vi "Analyse.vi"(8 "error in (no error)":errorcluster, 10 "ImageData":T1, 11 "AbsorptionAnalyser in":refnum<class "AbsorptionAnalyserNTU.lvclass">) -> (0 "error out":errorcluster, 3 "AbsorptionAnalyser out":refnum<class "AbsorptionAnalyserNTU.lvclass">)   [LabVIEW 2011, in "AbsorptionAnalyserNTU.lvclass"]
uses:
  AbsorptionAnalyserNTU.lvclass
  AbsorptionAnalyserNTU.lvclass/AbsorptionAnalyserNTU.ctl
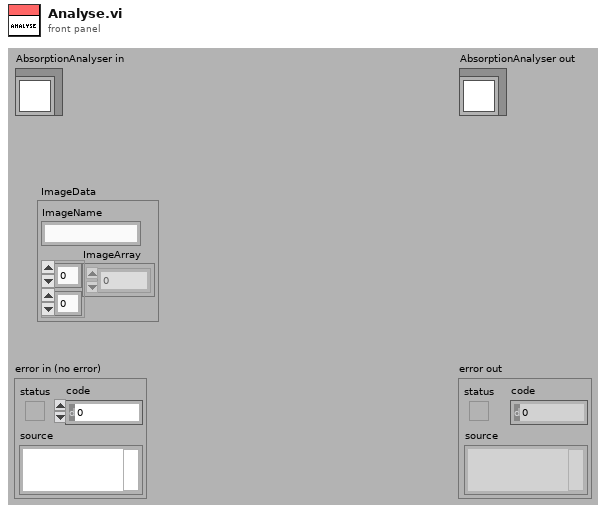
[diagram p1: front panel]
types:
  T1 = cluster{"ImageName":string, "ImageArray":sgl[][]}
  T2 = cluster{"ImageName":string, "ImageArray":sgl[][]}[]
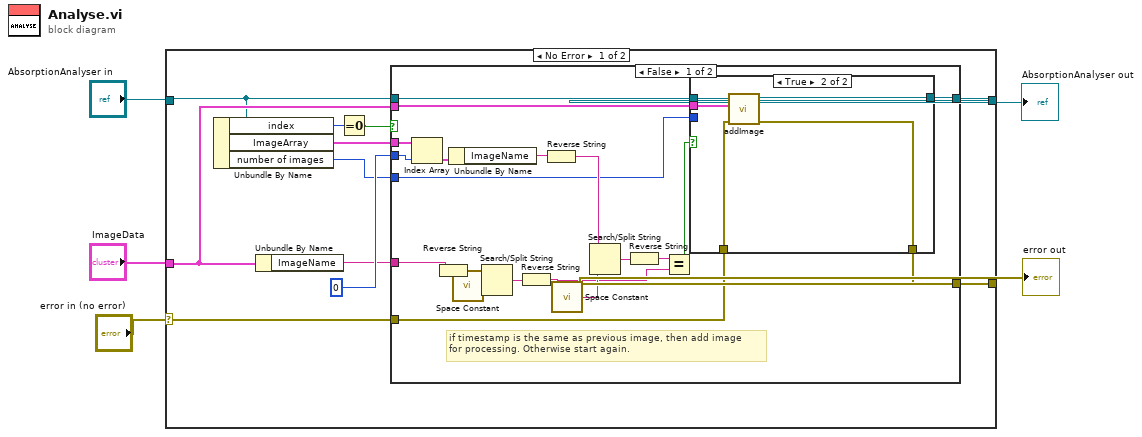
[diagram p0: block diagram]
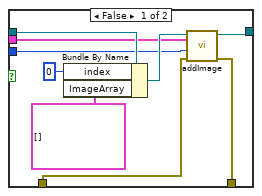
[diagram p2: hidden frame]
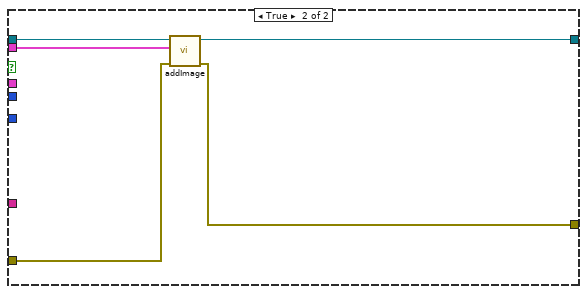
[diagram p3: hidden frame]
diagram:
  n1 = case shown="No Error" "error in (no error)" {
    selector: "error in (no error)" -> [w15 w56]
    tunnel: [w14 w56] -> w4
    tunnel: [w16 w57] -> w3
    tunnel: "AbsorptionAnalyser in" -> [w12 w57]
    tunnel: "ImageData" -> [w13 _]
    frame No Error {
      n2 = Unbundle By Name(w12) -> ("index"=w8:i32, "ImageArray"=w11:T2, "number of images"=w6:i32)
      n3 = Unbundle By Name(w13) -> ("ImageName"=w7:string)
      n4 = Equal To 0?(x=w8) -> (x = 0?=w9:bool)
      n5 = case shown="False" w9 {
        tunnel: [w21 w55] -> w16
        tunnel: w15 -> [w19 w54]
        tunnel: [w18 w53] -> w14
        tunnel: w13 -> [w20 w52]
        tunnel: w12 -> [w22 w51]
        tunnel: w11 -> [w35 _]
        tunnel: 0 -> [w36 _]
        tunnel: w7 -> [w26 _]
        tunnel: w6 -> [w17 _]
        frame False {
          # "if timestamp is the same as previous image, then add image\nfor processing. Otherwise start again."
          n6 = Index Array(array=w35, index=w36) -> (element=w34:T1)
          n7 = Reverse String(1:w26) -> (0:w29:string)
          n8 = Unbundle By Name(w34) -> ("ImageName"=w33:string)
          n9 = call <vilib>:"Space Constant.vi"() -> ("String"=w28:string)
          n10 = Search/Split String(string=w29, search string/char (-)=w28) -> (match + rest of string=w27:string)  [unwired: 1 in, 2 out]
          n11 = Reverse String(1:w27) -> (0:w24:string)
          n12 = Reverse String(1:w33) -> (0:w32:string)
          n13 = call <vilib>:"Space Constant.vi"() -> ("String"=w31:string)
          n14 = Search/Split String(string=w32, search string/char (-)=w31) -> (match + rest of string=w30:string)  [unwired: 1 in, 2 out]
          n15 = Reverse String(1:w30) -> (0:w25:string)
          n16 = Equal?(x=w25, y=w24) -> (x = y?=w23:bool)
          n17 = case shown="True" w23 {
            tunnel: w22 -> [w44 w50]
            tunnel: [w42 w49] -> w21
            tunnel: w20 -> [w40 w48]
            tunnel: w19 -> [w39 w47]
            tunnel: [w38 w46] -> w18
            tunnel: w17 -> [w37 _]
            frame False {
              n18 = Bundle By Name(cluster=w44, "index"=0, "ImageArray"=T2 []) -> (w43:refnum<class "AbsorptionAnalyserNTU.lvclass">)
              n19 = call "addImage.vi"("error in (no error)"=w39, "number of images"=w37, "ImageData"=w40, "AbsorptionAnalyser in"=w43) -> ("error out"=w38:errorcluster, "AbsorptionAnalyser out"=w42:refnum<class "AbsorptionAnalyserNTU.lvclass">)  [unwired: 6 in]
            }
            frame True {
              n20 = call "addImage.vi"("error in (no error)"=w47, "ImageData"=w48, "AbsorptionAnalyser in"=w50) -> ("error out"=w46:errorcluster, "AbsorptionAnalyser out"=w49:refnum<class "AbsorptionAnalyserNTU.lvclass">)  [unwired: 7 in]
            }
          }
        }
        frame True {
          n21 = call "addImage.vi"("error in (no error)"=w54, "ImageData"=w52, "AbsorptionAnalyser in"=w51) -> ("error out"=w53:errorcluster, "AbsorptionAnalyser out"=w55:refnum<class "AbsorptionAnalyserNTU.lvclass">)  [unwired: 7 in]
        }
      }
    }
    frame Error {
    }
  }
  "error out" <- w4
  "AbsorptionAnalyser out" <- w3
